vi "TMCM351-getActualPosition.vi"(3 "错误输入":errorcluster caption="错误输入（无错误）", 4 "motor":u8(ring) items=["x", "y", "z"], 5 "com in":refnum<visa-resource-name>) -> (0 "错误输出":errorcluster, 1 "Pisotion":i32, 2 "com out":refnum<visa-resource-name>)   [LabVIEW 2018]
uses:
  module_param.vi
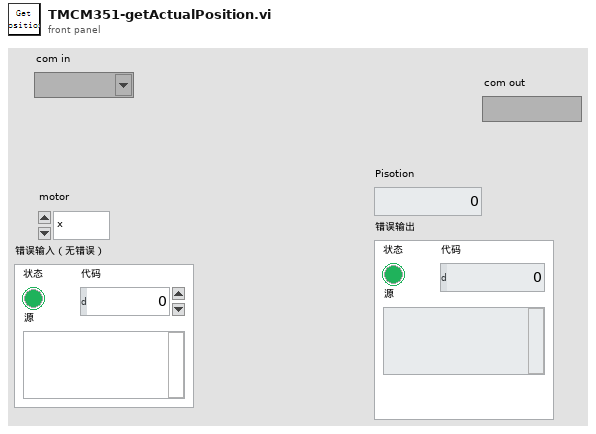
[diagram p1: front panel]
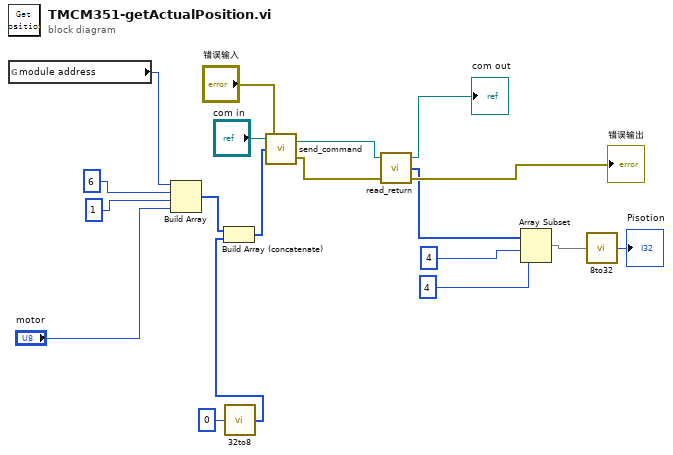
[diagram p0: block diagram]
diagram:
  n1 = global read "module_param.vi" "module address"() -> (w16:u8)
  n2 = Build Array(w16, u8 6, u8 1, "motor") -> (w14:u8[])
  n3 = call "32to8.vi"("32data_in"=0) -> ("8Array"=w13:u8[])
  n4 = Build Array (concatenate)(w14, w13) -> (w12:u8[])
  n5 = call "send_command.vi"("错误输入"="错误输入", 3:w12, "com in"="com in") -> ("错误输出"=w9:errorcluster, "com out"=w10:refnum<visa-resource-name>)
  n6 = call "read_return.vi"("错误输入（无错误）"=w9, "com in"=w10) -> ("错误输出"=→"错误输出":errorcluster, "return out"=w5:u8[], "com out"=→"com out":refnum<visa-resource-name>)  [unwired: 1 in]
  n7 = Array Subset(array=w5, index=4 ("索引"), length=4 ("长度")) -> (w2:u8[])
  n8 = call "8to32.vi"("Arrayin"=w2) -> ("data32"=→"Pisotion":i32)
